vi "UWB Serial Read.vi"(8 "Timeout (ms)":i32=-1, 9 "Bytes to Read":u32, 10 "FPGA VI Reference In":refnum<k20>, 11 "error in (no error)":errorcluster) -> (0 "String":string, 1 "Timeout?":bool, 2 "FPGA VI Reference Out":refnum<k20>, 3 "error out":errorcluster)   [LabVIEW 2016]
uses:
  <vilib>/rvi/errors/niLvFpgaAdjustHostInterfaceError.vi
  <vilib>/rvi/interface/nirviReadWriteControl/nirviReadWriteControl.xnode
  <vilib>/rvi/interface/Simulation/niFpgaSimulationCallBeginRW.vi
  NiFpgaLv.dll
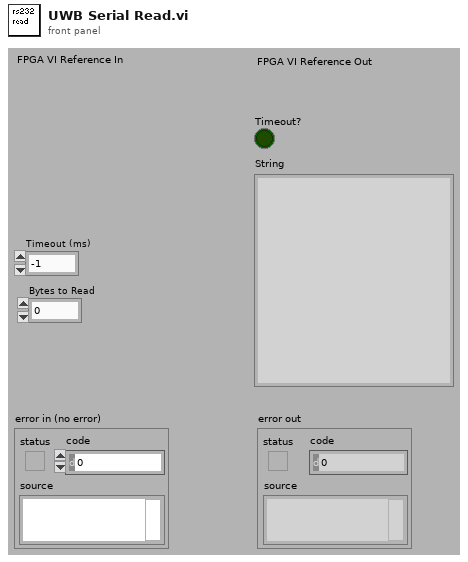
[diagram p1: front panel]
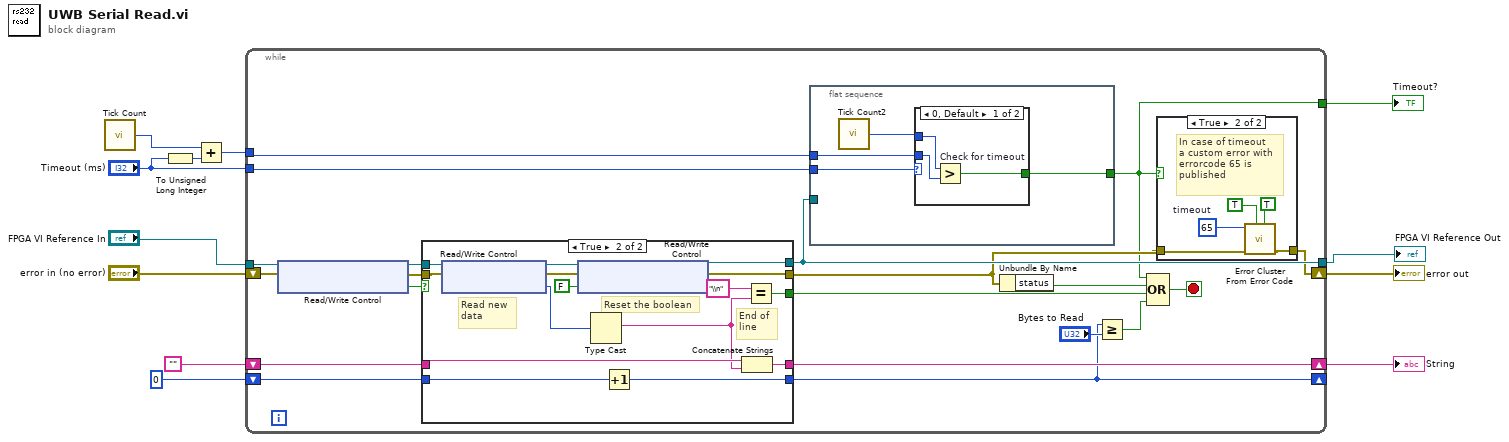
[diagram p0: block diagram]
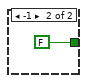
[diagram p3: hidden frame]
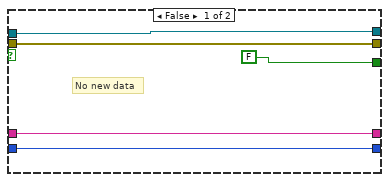
[diagram p4: hidden frame]
diagram:
  n1 = call "Tick Count"() -> ("Tick Count(mSec)"=w6:u32)
  n2 = To Unsigned Long Integer(number="Timeout (ms)") -> (unsigned 32bit integer=w3:u32)
  n3 = Add(x=w6, y=w3) -> (x+y=w7:u32)
  n4 = while {
    tunnel: "FPGA VI Reference In" -> [w26]
    tunnel: [w24] -> w1
    shift-right: [w23] -> _
    shift-left: u32 0 -> [w30]
    shift-right: [w28] -> w8
    shift-left: "" -> [w29]
    shift-right: [w15] -> w11
    shift-left: "error in (no error)" -> [w32]
    tunnel: "Timeout (ms)" -> [w20]
    tunnel: w7 -> [w19]
    tunnel: [w13] -> w5
    stop <- w22 stop-if-true
    n5 = xnode "Read/Write Control"("FPGA VI Reference In"=w26, "error in"=w32) -> ("FPGA VI Reference Out"=w25:refnum<k20>, "error out"=w18:errorcluster, "Read: New UWB Data"=w31:bool)
    n6 = case shown="True" w31 {
      tunnel: [w51 w66] -> w23
      tunnel: w30 -> [w51 w65]
      tunnel: w29 -> [w50 w64]
      tunnel: [w50 w63] -> w28
      tunnel: w25 -> [w49 w61]
      tunnel: [w49 w59] -> w24
      tunnel: [FALSE w58] -> w21
      tunnel: w18 -> [w47 w56]
      tunnel: [w47 w54] -> w17
      frame False {
        # "No new data"
      }
      frame True {
        # "End of \nline"
        # "Reset the boolean"
        # "Read new \ndata"
        n7 = xnode "Read/Write Control"("FPGA VI Reference In"=w61, "error in"=w56) -> ("FPGA VI Reference Out"=w60:refnum<k20>, "error out"=w55:errorcluster, "Read: UWB Char"=w62:u8)
        n8 = xnode "Read/Write Control"("FPGA VI Reference In"=w60, "error in"=w55, "Read: New UWB Data"=FALSE ("Data Read")) -> ("FPGA VI Reference Out"=w59:refnum<k20>, "error out"=w54:errorcluster)
        n9 = Type Cast(x=w62) -> (*(type *) &x=w57:string)  [unwired: 1 out]
        n10 = Increment(x=w65) -> (x+1=w66:u32)
        n11 = Concatenate Strings(w64, w57) -> (w63:string)
        n12 = Equal?(x="\\n", y=w57) -> (x = y?=w58:bool)
      }
    }
    n13 = flat-sequence {
      tunnel: w24 -> [_]
      tunnel: [w42] -> w13
      tunnel: w20 -> [w41]
      tunnel: w19 -> [w40]
      frame #0 {
        n14 = call "Tick Count2"() -> ("Tick Count(mSec)"=w39:u32)
        n15 = case shown="0, Default" w41 {
          tunnel: [w43 FALSE] -> w42
          tunnel: w40 -> [w44 _]
          tunnel: w39 -> [w45 _]
          frame 0, Default {
            n16 = Greater? "Check for timeout"(x=w45, y=w44) -> (0:w43:bool)
          }
          frame -1 {
          }
        }
      }
    }
    n17 = Unbundle By Name(w17) -> ("status"=w16:bool)
    n18 = Greater Or Equal?(x=w23, y="Bytes to Read") -> (x >= y?=w14:bool)
    n19 = Compound Arithmetic op=OR(w13, w16, w21, w14) -> (w22:bool)
    n20 = case shown="True" w13 {
      tunnel: w17 -> [w33 w37]
      tunnel: [w33 w36] -> w15
      frame False {
      }
      frame True {
        w38 = 65  # timeout
        # "In case of timeout\na custom error with\nerrorcode 65 is \npublished"
        n21 = call <vilib>:"Error Cluster From Error Code.vi"("is warning? (False)"=TRUE, "show call chain? (False)"=TRUE, "error in (no error)"=w37, "error code (0)"=w38) -> ("error out"=w36:errorcluster)  [unwired: 5 out]
      }
    }
  }
  "error out" <- w11
  "String" <- w8
  "Timeout?" <- w5
  "FPGA VI Reference Out" <- w1
